vi "0037-0007.vi"() -> ()   [LabVIEW 2014]
panel:
  in  "アプリ終了":bool
  in  "全データ保存":bool
  in  "停止ボタン":bool
  in  "測定間隔（秒）":dbl=5.0 min=5.0 step=5.0
  in  "再生ボタン":bool
  out "８":bool
  out "７":bool
  out "６":bool
  out "５":bool
  out "４":bool
  out "３":bool
  out "２":bool
  out "１":bool
  in  "?":T1(tab)
  out "Temp.":cluster{dbl[], dbl[]}[](graph)
  out "Humi.":cluster{dbl[], dbl[]}[](graph)
  out "Temp. 1":cluster{dbl[], dbl[]}(graph)
  out "Humi. 1":cluster{dbl[], dbl[]}(graph)
  out "Temp. 2":cluster{dbl[], dbl[]}(graph)
  out "Humi. 2":cluster{dbl[], dbl[]}(graph)
  out "Temp. 3":cluster{dbl[], dbl[]}(graph)
  out "Humi. 3":cluster{dbl[], dbl[]}(graph)
  out "Temp. 4":cluster{dbl[], dbl[]}(graph)
  out "Humi. 4":cluster{dbl[], dbl[]}(graph)
  out "Temp. 5":cluster{dbl[], dbl[]}(graph)
  out "Humi. 5":cluster{dbl[], dbl[]}(graph)
  out "Temp. 6":cluster{dbl[], dbl[]}(graph)
  out "Humi. 6":cluster{dbl[], dbl[]}(graph)
  out "Temp. 7":cluster{dbl[], dbl[]}(graph)
  out "Humi. 7":cluster{dbl[], dbl[]}(graph)
  out "Temp. 8":cluster{dbl[], dbl[]}(graph)
  out "Humi. 8":cluster{dbl[], dbl[]}(graph)
  out "停止報告":bool
  out "開始合図":bool
  out "停止合図":bool
  out "温湿度データ 2":dbl[][](array[numeric])
  out "稼働状態":bool
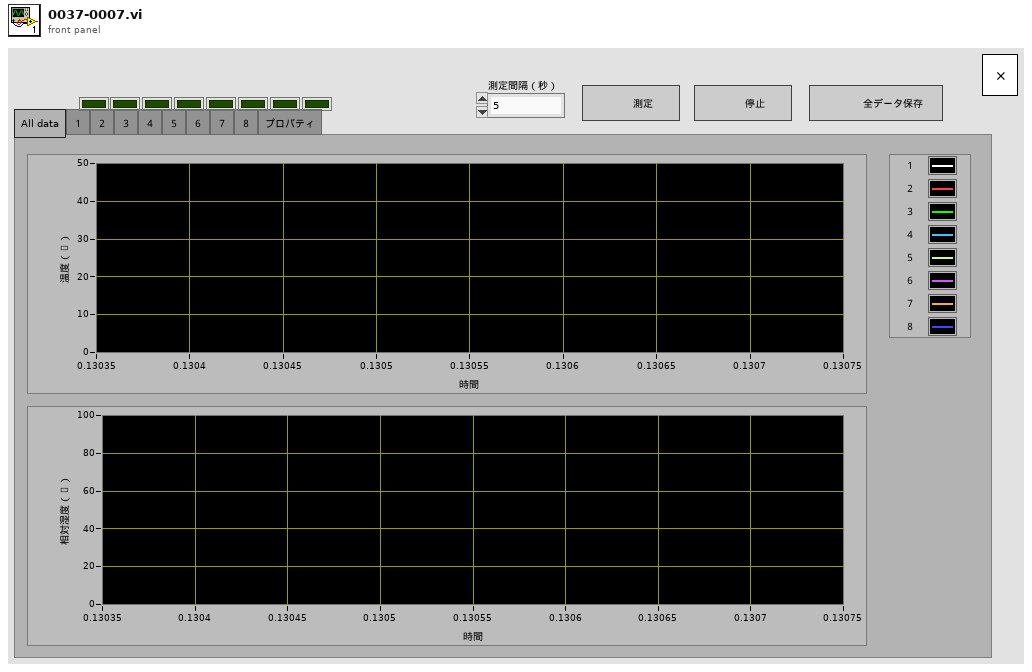
[diagram p1: front panel]
types:
  T1 = enum32{"All data", "１", "２", "３", "４", "５", "６", "７", "８", "プロパティ"}
  T2 = cluster{"bitRate":u32, "address":u8, "autoReadRespond":bool, "writeTimeout":u16, "readTimeout":u16, "sclLowTimeout":bool, "transferRetries":u16}
  T3 = typedef "CP2112_device.ctl" = i32
  T4 = cluster{cluster{dbl[], dbl[]}, cluster{dbl[], dbl[]}, cluster{dbl[], dbl[]}, cluster{dbl[], dbl[]}, cluster{dbl[], dbl[]}, cluster{dbl[], dbl[]}, cluster{dbl[], dbl[]}, cluster{dbl[], dbl[]}, cluster{dbl[], dbl[]}}
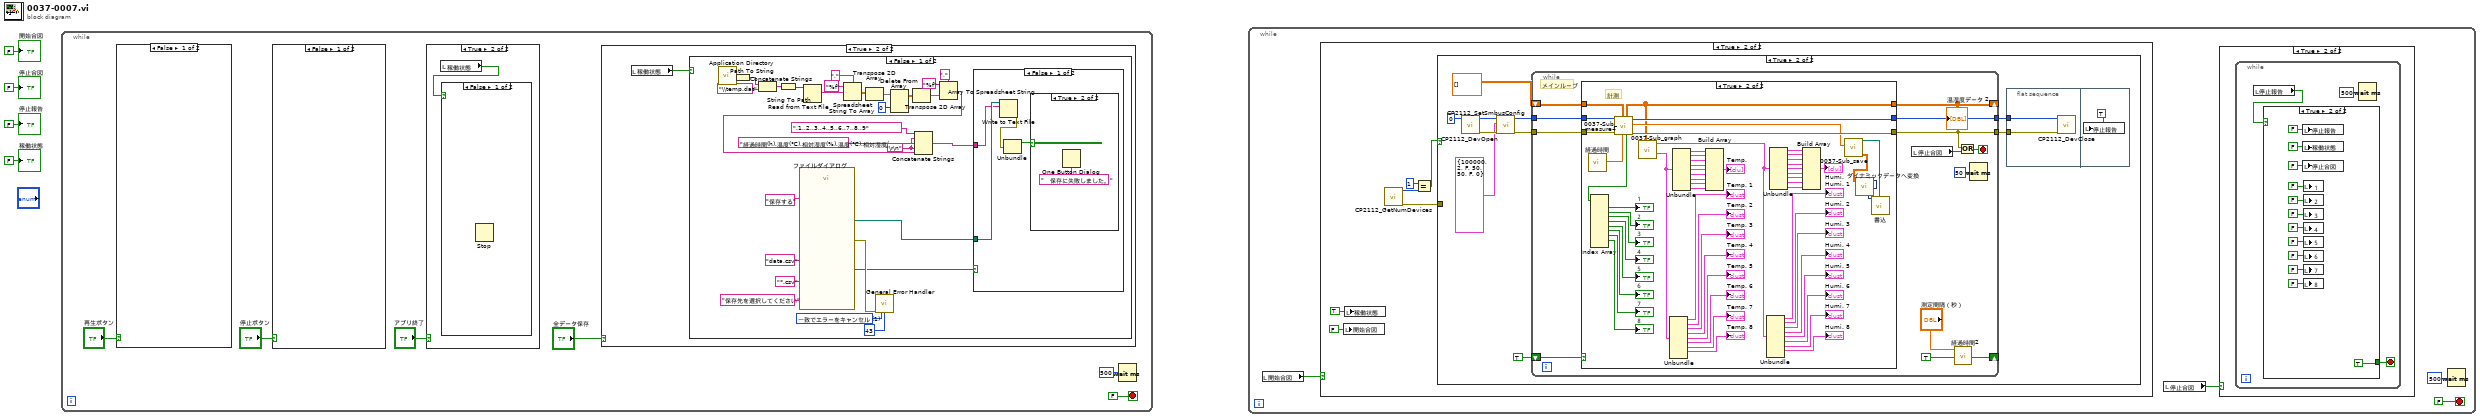
[diagram p0: block diagram]
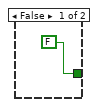
[diagram p3: hidden frame]
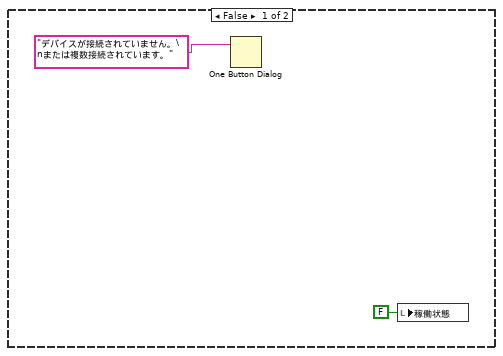
[diagram p5: hidden frame]
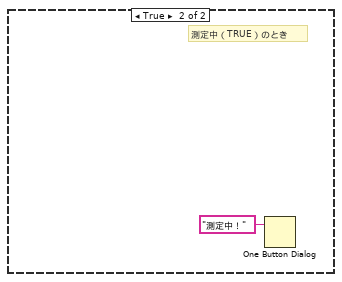
[diagram p10: hidden frame]
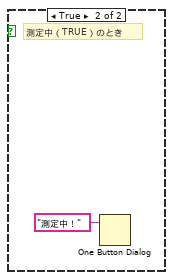
[diagram p12: hidden frame]
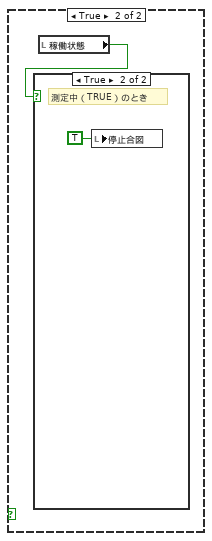
[diagram p13: hidden frame]
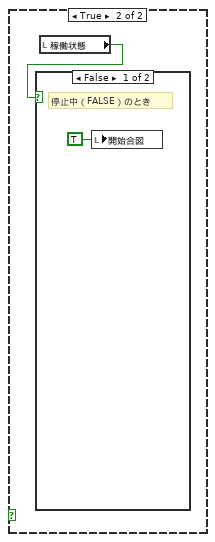
[diagram p15: hidden frame]
diagram:
  n1 = while {
    stop <- FALSE stop-if-true
    n2 = case shown="FALSE" "再生ボタン" {
      frame False {
      }
      frame True {
        n3 = local read "稼働状態"() -> (w51:bool)
        n4 = case shown="FALSE" w51 {
          frame False {
            # "停止中（FALSE）のとき"
            n5 = local write "開始合図"(TRUE ("測定開始")) -> ()
          }
          frame True {
          }
        }
      }
    }
    n6 = case shown="FALSE" "停止ボタン" {
      frame False {
      }
      frame True {
        n7 = local read "稼働状態"() -> (w49:bool)
        n8 = case shown="TRUE" w49 {
          frame False {
          }
          frame True {
            # "測定中（TRUE）のとき"
            n9 = local write "停止合図"(TRUE ("測定開始")) -> ()
          }
        }
      }
    }
    n10 = case shown="TRUE" "アプリ終了" {
      frame False {
      }
      frame True {
        n11 = local read "稼働状態"() -> (w47:bool)
        n12 = case shown="FALSE" w47 {
          frame False {
            n13 = Stop() -> ()  [unwired: 1 in]
          }
          frame True {
            # "測定中（TRUE）のとき"
            n14 = One Button Dialog(message="測定中！" ("メッセージ")) -> ()  [unwired: 1 in, 1 out]
          }
        }
      }
    }
    n15 = case shown="TRUE" "全データ保存" {
      frame False {
      }
      frame True {
        n16 = local read "稼働状態"() -> (w11:bool)
        n17 = case shown="FALSE" w11 {
          frame False {
            w13 = "\r\n"
            w31 = 1 items=["例外なし", "一致でエラーをキャンセル", "一致でエラーをセット"] ("[exception action] (none:0)")
            n18 = call <vilib>:"Application Directory.vi"() -> ("Application Directory"=w39:path)
            n19 = Path To String(path=w39) -> (string=w38:string)
            n20 = Concatenate Strings(w38, "\\temp.dat" ("文字列")) -> (w37:string)
            n21 = String To Path(string=w37) -> (path=w36:path)
            n22 = call "ファイルダイアログ"("prompt"="保存先を選択してください", "button label"="保存する", "default name"="data.csv", "pattern (all files)"="*.csv") -> ("selected path"=w28:path, "cancelled"=w27:bool, "error out"=w29:errorcluster)  [unwired: 8 in, 1 out]
            n23 = Read from Text File(file (use dialog)=w36) -> (text=w26:string)  [unwired: 3 in, 3 out]
            n24 = Spreadsheet String To Array(delimiter (Tab)="," ("デリミタ（タブ）"), format string="%f" ("形式文字列"), spreadsheet string=w26) -> (array=w17:dbl[][])  [unwired: 1 in]
            n25 = Transpose 2D Array(2D array=w17) -> (transposed array=w23:dbl[][])
            n26 = call <vilib>:"General Error Handler.vi"("error in (no error)"=w29, "[exception action] (none:0)"=w31, "[exception code]"=43) -> ()  [unwired: 8 in, 5 out]
            n27 = Delete From Array(array=w23, index (row)=0 ("指標 （行）")) -> (array with subset deleted=w21:dbl[][])  [unwired: 2 in, 1 out]
            n28 = Transpose 2D Array(2D array=w21) -> (transposed array=w20:dbl[][])
            n29 = Array To Spreadsheet String(delimiter (Tab)="," ("デリミタ（タブ）"), array=w20, 3:"%f" ("形式文字列")) -> (spreadsheet string=w15:string)
            n30 = Concatenate Strings(",1,,2,,3,,4,,5,,6,,7,,8,,9", w13, "経過時間(h),温度(℃),相対湿度(%),温度(℃),相対湿度(%),温度(℃),相対湿度(%),温度(℃),相対湿度(%),温度(℃),相対湿度(%),温度(℃),相対湿度(%),温度(℃),相対湿度(%),温度(℃),相対湿度(%),温度(℃),相対湿度(%)", w13, w15) -> (w14:string)
            n31 = case shown="FALSE" w27 {
              tunnel: w28 -> [w44 _]
              tunnel: w14 -> [w41 _]
              frame False {
                n32 = Write to Text File(file (use dialog)=w44, text=w41) -> (error out=w43:errorcluster)  [unwired: 2 in, 2 out]
                n33 = Unbundle(w43) -> ("status"=w42:bool)  [unwired: 2 out]
                n34 = case shown="TRUE" w42 {
                  frame False {
                  }
                  frame True {
                    n35 = One Button Dialog(message="　保存に失敗しました。" ("メッセージ")) -> ()  [unwired: 1 in, 1 out]
                  }
                }
              }
              frame True {
              }
            }
          }
          frame True {
            # "測定中（TRUE）のとき"
            n36 = One Button Dialog(message="測定中！" ("メッセージ")) -> ()  [unwired: 1 in, 1 out]
          }
        }
      }
    }
    n37 = Wait (ms)(milliseconds to wait=u32 500 ("ミリ秒待機時間")) -> ()  [unwired: 1 out]
  }
  n38 = while {
    stop <- FALSE stop-if-true
    n39 = local read "開始合図"() -> (w54:bool)
    n40 = case shown="TRUE" w54 {
      frame False {
      }
      frame True {
        n41 = local write "開始合図"(FALSE ("測定開始")) -> ()
        n42 = local write "稼働状態"(TRUE ("稼働状態")) -> ()
        n43 = call "CP2112_GetNumDevices.vi"() -> ("error out"=w75:errorcluster, "numDevices"=w77:i32)  [unwired: 9 in, 1 out]
        n44 = Equal?(x=1, y=w77) -> (x = y?=w76:bool)
        n45 = case shown="TRUE" w76 {
          tunnel: w75 -> [_ _]
          frame False {
            n46 = One Button Dialog(message="デバイスが接続されていません。\nまたは複数接続されています。" ("メッセージ")) -> ()  [unwired: 1 in, 1 out]
            n47 = local write "稼働状態"(FALSE ("稼働状態")) -> ()
          }
          frame True {
            n48 = call "CP2112_DevOpen.vi"("deviceNum"=0) -> ("error out"=w85:errorcluster, "device"=w82:T3)  [unwired: 8 in, 1 out]
            n49 = call "CP2112_SetSmbusConfig.vi"("error in (no error)"=w85, "smbusInfo"=T2 {"bitRate"=100000, "address"=2, "autoReadRespond"=FALSE, "writeTimeout"=50, "readTimeout"=50, "sclLowTimeout"=FALSE, "transferRetries"=0}, "device"=w82) -> ("error out"=w84:errorcluster, "deviceOut"=w83:T3)  [unwired: 6 in, 1 out]
            n50 = while {
              tunnel: w84 -> [w105]
              tunnel: w83 -> [w104]
              tunnel: [w97] -> w90
              tunnel: [w103] -> w89
              shift-right: [w99] -> _
              shift-left: TRUE -> [w100]
              shift-right: [w94] -> _
              shift-left: dbl[][] [] ("温湿度データ") -> [w95]
              stop <- w96 stop-if-true
              # "メインループ"
              n51 = case shown="TRUE" w100 {
                tunnel: w105 -> [w109 w167]
                tunnel: w104 -> [w108 w166]
                tunnel: [w109 w155] -> w97
                tunnel: [w108 w156] -> w103
                tunnel: w95 -> [w107 w157]
                tunnel: [w107 w110] -> w94
                frame False {
                }
                frame True {
                  # "計測"
                  n52 = call "経過時間"() -> ("Elapsed Time (s)"=w153:dbl)  [unwired: 12 in, 7 out]
                  n53 = call "0037-Sub_measure4.vi"("数値"=w153, "温湿度データ"=w157, "error out"=w167, "device"=w166) -> ("error out 2"=w155:errorcluster, "出力配列"=w111:dbl[], "device 2"=w156:T3, "配列"=w154:bool[], "温湿度データ 2"=w110:dbl[][])  [unwired: 3 in]
                  n54 = Index Array(array=w154) -> (element #1=→"１":bool, element #2=→"２":bool, element #3=→"３":bool, element #4=→"４":bool, element #5=→"５":bool, element #6=→"６":bool, element #7=→"７":bool, element #8=→"８":bool)  [unwired: 9 in, 1 out]
                  n55 = call "0037-Sub_graph.vi"("温湿度データ"=w110) -> ("温度"=w149:T4, "湿度"=w132:T4)  [unwired: 9 in]
                  n56 = Unbundle(w149) -> (→"Temp. 1":cluster{dbl[], dbl[]}, →"Temp. 2":cluster{dbl[], dbl[]}, →"Temp. 3":cluster{dbl[], dbl[]}, →"Temp. 4":cluster{dbl[], dbl[]}, →"Temp. 5":cluster{dbl[], dbl[]}, →"Temp. 6":cluster{dbl[], dbl[]}, →"Temp. 7":cluster{dbl[], dbl[]}, →"Temp. 8":cluster{dbl[], dbl[]})  [unwired: 1 out]
                  n57 = Unbundle(w149) -> (w152:cluster{dbl[], dbl[]}, w151:cluster{dbl[], dbl[]}, w148:cluster{dbl[], dbl[]}, w147:cluster{dbl[], dbl[]}, w146:cluster{dbl[], dbl[]}, w145:cluster{dbl[], dbl[]}, w144:cluster{dbl[], dbl[]}, w143:cluster{dbl[], dbl[]}, w142:cluster{dbl[], dbl[]})
                  n58 = Build Array(w152, w151, w148, w147, w146, w145, w144, w143, w142) -> (→"Temp.":cluster{dbl[], dbl[]}[])
                  n59 = Unbundle(w132) -> (→"Humi. 1":cluster{dbl[], dbl[]}, →"Humi. 2":cluster{dbl[], dbl[]}, →"Humi. 3":cluster{dbl[], dbl[]}, →"Humi. 4":cluster{dbl[], dbl[]}, →"Humi. 5":cluster{dbl[], dbl[]}, →"Humi. 6":cluster{dbl[], dbl[]}, →"Humi. 7":cluster{dbl[], dbl[]}, →"Humi. 8":cluster{dbl[], dbl[]})  [unwired: 1 out]
                  n60 = Unbundle(w132) -> (w141:cluster{dbl[], dbl[]}, w140:cluster{dbl[], dbl[]}, w139:cluster{dbl[], dbl[]}, w138:cluster{dbl[], dbl[]}, w137:cluster{dbl[], dbl[]}, w136:cluster{dbl[], dbl[]}, w135:cluster{dbl[], dbl[]}, w134:cluster{dbl[], dbl[]}, w133:cluster{dbl[], dbl[]})
                  n61 = Build Array(w141, w140, w139, w138, w137, w136, w135, w134, w133) -> (→"Humi.":cluster{dbl[], dbl[]}[])
                  n62 = call "0037-Sub_save.vi"("部分配列 2"=w111) -> ("パス"=w114:path, "転置配列"=w112:dbl[][])  [unwired: 8 in]
                  n63 = call "ダイナミックデータへ変換"("2D Array"=w112) -> ("Dynamic Data Type"=w113:dynamicdata)  [unwired: 3 in]
                  n64 = call "書込"("Signals"=w113, "Filename"=w114) -> ()  [unwired: 15 in, 3 out]
                }
              }
              "温湿度データ 2" <- w94
              n65 = local read "停止合図"() -> (w98:bool)
              n66 = call "経過時間2"("Time Target (s)"="測定間隔（秒）", "Auto Reset"=TRUE) -> ("Time has Elapsed"=w99:bool)  [unwired: 10 in, 7 out]
              n67 = Or(x=w97, y=w98) -> (x .or. y?=w96:bool)
              n68 = Wait (ms)(milliseconds to wait=u32 50 ("ミリ秒待機時間")) -> ()  [unwired: 1 out]
            }
            n69 = flat-sequence {
              tunnel: w90 -> [w92]
              tunnel: w89 -> [w91]
              frame #0 {
                n70 = call "CP2112_DevClose.vi"("error in (no error)"=w92, "device"=w91) -> ()  [unwired: 9 in, 1 out]
              }
              frame #1 {
                n71 = local write "停止報告"(TRUE ("停止報告")) -> ()
              }
            }
          }
        }
      }
    }
    n72 = local read "停止合図"() -> (w53:bool)
    n73 = case shown="TRUE" w53 {
      frame False {
      }
      frame True {
        n74 = while {
          stop <- w57 stop-if-true
          n75 = local read "停止報告"() -> (w59:bool)
          n76 = case shown="TRUE" w59 {
            tunnel: [FALSE TRUE] -> w57
            frame False {
            }
            frame True {
              n77 = local write "停止報告"(FALSE ("停止報告")) -> ()
              n78 = local write "稼働状態"(FALSE ("稼働状態")) -> ()
              n79 = local write "停止合図"(FALSE ("停止合図")) -> ()
              n80 = local write "１"(FALSE ("１")) -> ()
              n81 = local write "２"(FALSE ("２")) -> ()
              n82 = local write "３"(FALSE ("３")) -> ()
              n83 = local write "４"(FALSE ("４")) -> ()
              n84 = local write "５"(FALSE ("５")) -> ()
              n85 = local write "６"(FALSE ("６")) -> ()
              n86 = local write "７"(FALSE ("７")) -> ()
              n87 = local write "８"(FALSE ("８")) -> ()
            }
          }
          n88 = Wait (ms)(milliseconds to wait=u32 500 ("ミリ秒待機時間")) -> ()  [unwired: 1 out]
        }
      }
    }
    n89 = Wait (ms)(milliseconds to wait=u32 500 ("ミリ秒待機時間")) -> ()  [unwired: 1 out]
  }
  "開始合図" <- FALSE ("測定開始")
  "停止合図" <- FALSE ("測定停止")
  "稼働状態" <- FALSE ("稼働状態")
  "停止報告" <- FALSE ("停止報告")
